vi "Sent_Recive.vi"(4 "帧长度":u8, 5 "CAN_FRAME":T3, 6 "wait for reply (T)":bool=TRUE, 7 "帧格式":u8(ring) items=["数据帧", "远程帧"], 8 "error in (no error)":errorcluster, 9 "帧类型":u8(ring) items=["标准帧", "扩展帧"], 10 "ID":u32) -> (0 "error out":errorcluster, 1 "timed out?":bool, 2 "Reply Payload":T1)   [LabVIEW 2020, in "ZLG_CAN.lvlib"]
doc: "_____\nCreated using Delacor QMH Event Scripter 4.2.1.88."
uses:
  ZLG_CAN.lvlib
  CAN_Frame.ctl
  Sent_Recive (Reply Payload)--cluster.ctl
  CAN_OBJ_R.ctl
  Sent_Recive Argument--cluster.ctl
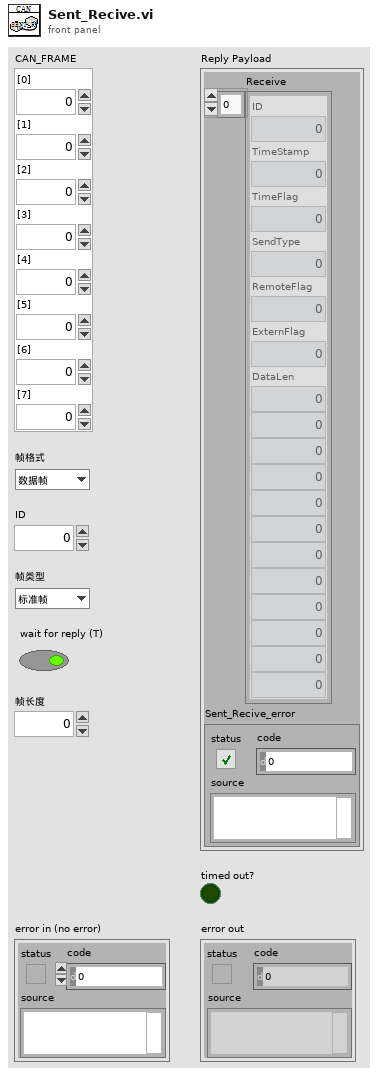
[diagram p1: front panel]
types:
  T1 = typedef "ZLG_CAN.lvlib/Sent_Recive (Reply Payload)--cluster.ctl" = cluster{"Receive":T2[], "Sent_Recive_error":errorcluster}
  T2 = typedef "ZLG_CAN.lvlib/CAN_OBJ_R.ctl" = cluster{"ID":u32, "TimeStamp":u32, "TimeFlag":u8, "SendType":u8, "RemoteFlag":u8, "ExternFlag":u8, "DataLen":u8, "数值":u8, "数值":u8, "数值":u8, "数值":u8, "数值":u8, "数值":u8, "数值":u8, "数值":u8, "数值":u8, "数值":u8, "数值":u8}
  T3 = typedef "ZLG_CAN.lvlib/CAN_Frame.ctl" = cluster{"[0]":u8, "[1]":u8, "[2]":u8, "[3]":u8, "[4]":u8, "[5]":u8, "[6]":u8, "[7]":u8}
  T4 = typedef "ZLG_CAN.lvlib/Sent_Recive Argument--cluster.ctl" = cluster{"ID":u32, "帧类型":u8, "帧格式":u8, "CAN_FRAME":T3, "帧长度":u8, "Wait Notifier":refnum<notifier>, "wait for reply":bool}
  T5 = typedef "ZLG_CAN.lvlib/Request Events--cluster.ctl" = cluster{"Stop Module":refnum<user-event>, "Show Panel":refnum<user-event>, "Hide Panel":refnum<user-event>, "Get Module Execution Status":refnum<user-event>, "Show Diagram":refnum<user-event>, "Open_CAN":refnum<user-event>, "Init_CAN":refnum<user-event>, "Start_CAN":refnum<user-event>, "Sent_CAN":refnum<user-event>, "Close_CAN":refnum<user-event>, "Reset_CAN":refnum<user-event>, "Recive_CAN":refnum<user-event>, "Recive_Wait":refnum<user-event>, "Sent_Recive":refnum<user-event>}
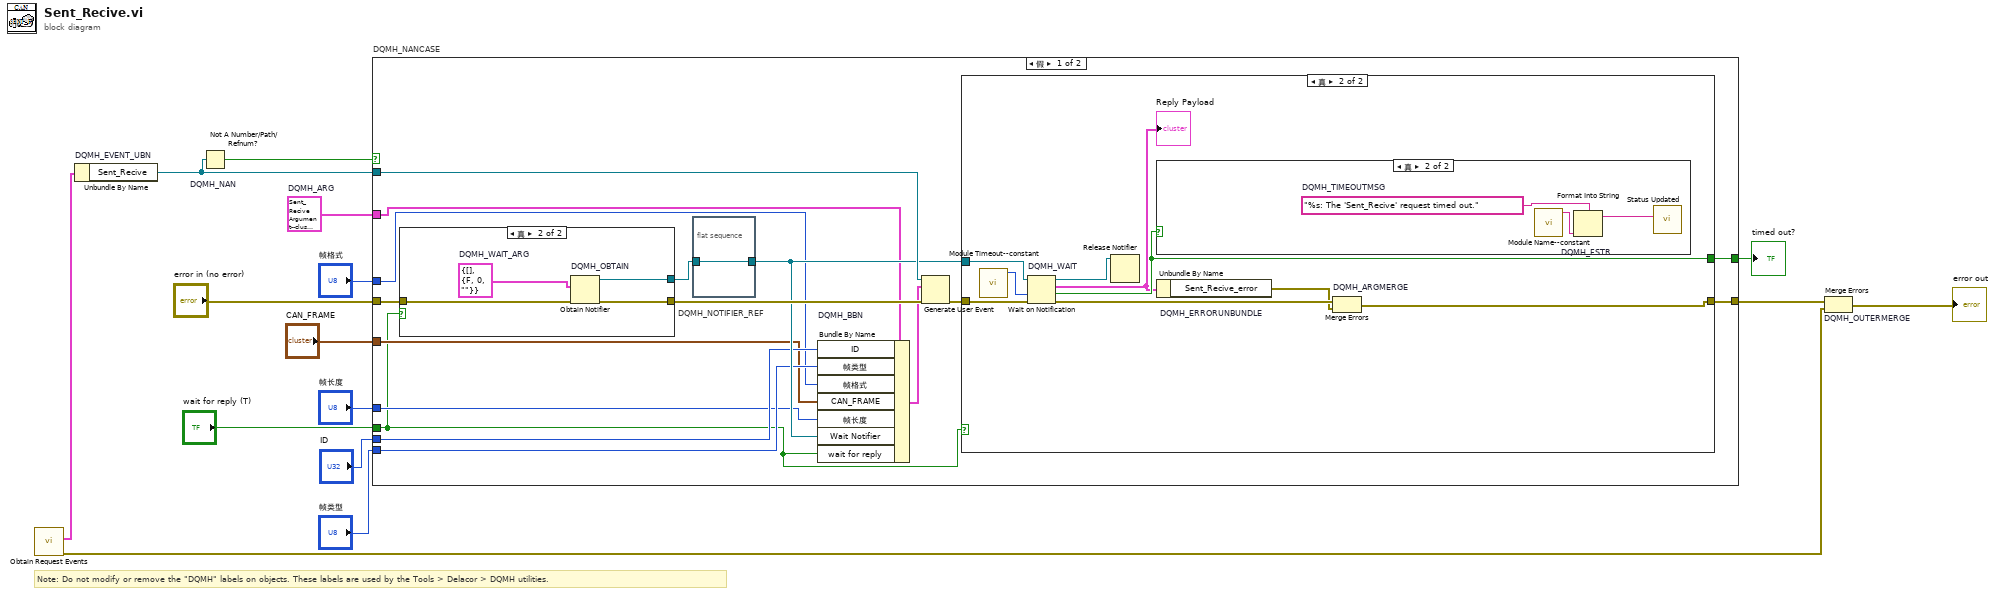
[diagram p0: block diagram]
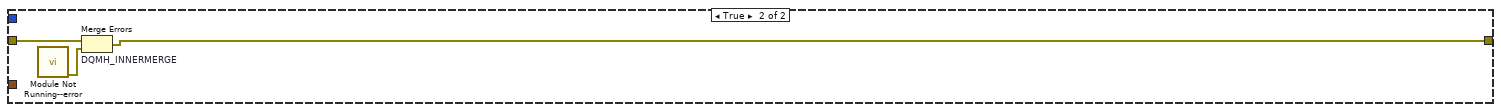
[diagram p5: hidden frame]
diagram:
  w9 = T4 {"ID"=0, "帧类型"=0, "帧格式"=0, "CAN_FRAME"={"[0]"=0, "[1]"=0, "[2]"=0, "[3]"=0, "[4]"=0, "[5]"=0, "[6]"=0, "[7]"=0}, "帧长度"=0, "Wait Notifier"=refnum, "wait for reply"=FALSE}  # DQMH_ARG
  # "Note: Do not modify or remove the \"DQMH\" labels on objects. These labels are used by the Tools > Delacor > DQMH utilities."
  n1 = call "Obtain Request Events.vi"() -> ("error out"=w2:errorcluster, "ZLG_CAN Request Events"=w1:T5)  [unwired: 10 in]
  n2 = Unbundle By Name "DQMH_EVENT_UBN"(w1) -> ("Sent_Recive"=w13:refnum<user-event>)
  n3 = Not A Number/Path/Refnum? "DQMH_NAN"(number/path/refnum=w13) -> (NaN/Path/Refnum?=w12:bool)
  n4 = case "DQMH_NANCASE" shown="假" w12 {
    tunnel: "error in (no error)" -> [w31 w53]
    tunnel: w13 -> [w29 _]
    tunnel: [w26 w52] -> w10
    tunnel: [w27 _] -> w11
    tunnel: w9 -> [w22 _]
    tunnel: "ID" -> [w21 _]
    tunnel: "帧类型" -> [w20 _]
    tunnel: "帧格式" -> [w19 _]
    tunnel: "CAN_FRAME" -> [w18 _]
    tunnel: "帧长度" -> [w17 _]
    tunnel: "wait for reply (T)" -> [w16 _]
    frame False {
      n5 = case shown="真" w16 {
        tunnel: w31 -> [w46 w50]
        tunnel: [w46 w49] -> w28
        tunnel: [_ w47] -> w24
        frame False {
        }
        frame True {
          w48 = T1 {"Receive"=[], "Sent_Recive_error"={"status"=FALSE, "code"=0, "source"=""}}  # DQMH_WAIT_ARG
          n6 = Obtain Notifier "DQMH_OBTAIN"(notification data type=w48, error in (no error)=w50) -> (notifier out=w47:refnum<notifier>, error out=w49:errorcluster)  [unwired: 2 in, 1 out]
        }
      }
      n7 = flat-sequence "DQMH_NOTIFIER_REF" {
        tunnel: w24 -> [w32]
        tunnel: [w32] -> w23
        frame #0 {
        }
      }
      n8 = Bundle By Name "DQMH_BBN"(cluster=w22, "ID"=w21, "帧类型"=w20, "帧格式"=w19, "CAN_FRAME"=w18, "帧长度"=w17, "Wait Notifier"=w23, "wait for reply"=w16) -> (w25:T4)
      n9 = Generate User Event(user event=w29, event data cluster=w25, error in=w28) -> (error out=w30:errorcluster)  [unwired: 1 in, 1 out]
      n10 = case "条件结构" shown="真" w16 {
        tunnel: w30 -> [w33 w42]
        tunnel: w23 -> [_ w40]
        tunnel: [_ w38] -> w27
        tunnel: [w33 w37] -> w26
        frame False {
        }
        frame True {
          n11 = call "Module Timeout--constant.vi"() -> ("Module Timeout"=w34:i32)  [unwired: 11 in]
          n12 = Wait on Notification "DQMH_WAIT"(notifier=w40, timeout in ms (-1)=w34, error in (no error)=w42) -> (notifier out=w39:refnum<notifier>, notification=w35:T1, timed out?=w38:bool, error out=w41:errorcluster)  [unwired: 1 in]
          "Reply Payload" <- w35
          n13 = Release Notifier ("释放通知器引用")(notifier=w39) -> ()  [unwired: 2 in, 3 out]
          n14 = case "条件结构" shown="真" w38 {
            frame False {
            }
            frame True {
              w45 = "%s: The 'Sent_Recive' request timed out."  # DQMH_TIMEOUTMSG
              n15 = call "Module Name--constant.vi"() -> ("Module Name"=w44:string)  [unwired: 11 in]
              n16 = Format Into String "DQMH_FSTR"(format string=w45, w44) -> (resulting string=w43:string)  [unwired: 2 in, 1 out]
              n17 = call "Status Updated.vi"("Status"=w43) -> ()  [unwired: 10 in, 1 out]
            }
          }
          n18 = Unbundle By Name "DQMH_ERRORUNBUNDLE"(w35) -> ("Sent_Recive_error"=w36:errorcluster)
          n19 = Merge Errors "DQMH_ARGMERGE"(w41, w36) -> (w37:errorcluster)
        }
      }
    }
    frame True {
      n20 = call "Module Not Running--error.vi"() -> ("error out"=w51:errorcluster)  [unwired: 11 in]
      n21 = Merge Errors "DQMH_INNERMERGE"(w53, w51) -> (w52:errorcluster)
    }
  }
  "timed out?" <- w11
  n22 = Merge Errors "DQMH_OUTERMERGE"(w10, w2) -> (→"error out":errorcluster)
